vi "WireReadBlockDiagram.vi"(8 "error in":errorcluster, 10 "Terminal References":T3, 11 "State":T1={"paths"={"index cluster path"=path "C:/Users/bcelis.AMER/Documents/TBDCore/source/Utilities/Cluster to Tag Bus Scripts/Controls/IndexCluster.ctl", "cluster path"=path "C:/Users/bcelis.AMER/Documents/TBDCore/source/Utilities/Cluster to Tag Bus Scripts/Controls/SampleControl.ctl", "cluster to tag bus VI path"=path "C:/Users/bcelis.AMER/Documents/TBDCore/source/Utilities/Cluster to Tag Bus Scripts/ClustertoTagbus.vi", " tag bus to cluster VI path"=path ""}, "write VI ref"=refnum, "read VI ref"=refnum, "base cluster"=variant}) -> (0 "error out":errorcluster, 3 "State out":T1={"paths"={"index cluster path"=path "C:/Users/bcelis.AMER/Documents/TBDCore/source/Utilities/Cluster to Tag Bus Scripts/Controls/IndexCluster.ctl", "cluster path"=path "C:/Users/bcelis.AMER/Documents/TBDCore/source/Utilities/Cluster to Tag Bus Scripts/Controls/SampleControl.ctl", "cluster to tag bus VI path"=path "C:/Users/bcelis.AMER/Documents/TBDCore/source/Utilities/Cluster to Tag Bus Scripts/ClustertoTagbus.vi", " tag bus to cluster VI path"=path ""}, "write VI ref"=refnum, "read VI ref"=refnum, "base cluster"=variant})   [LabVIEW 2013]
uses:
  Controls/TerminalReferences.ctl
  Controls/StateCluster.ctl
  Controls/PathsCluster.ctl
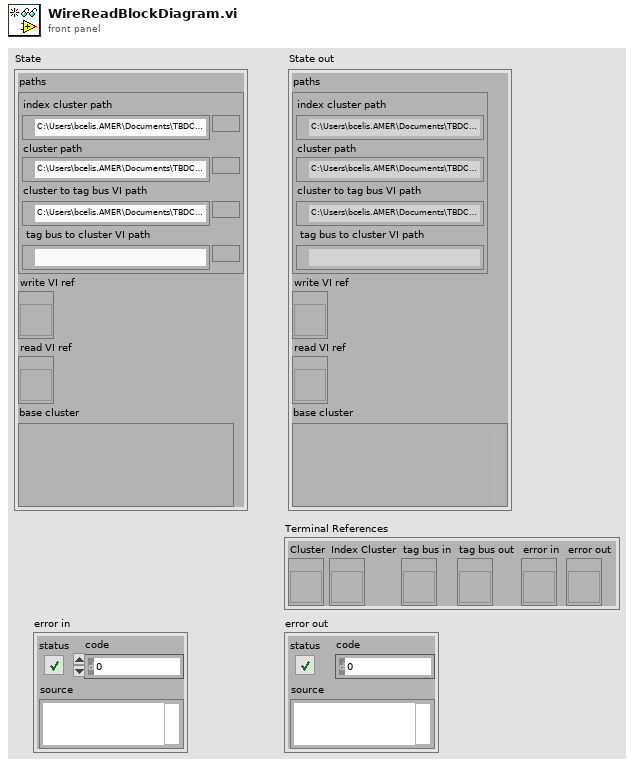
[diagram p1: front panel]
types:
  T1 = typedef "StateCluster.ctl" = cluster{"paths":T2, "write VI ref":refnum<vi>, "read VI ref":refnum<vi>, "base cluster":variant}
  T2 = typedef "PathsCluster.ctl" = cluster{"index cluster path":path, "cluster path":path, "cluster to tag bus VI path":path, " tag bus to cluster VI path":path}
  T3 = typedef "TerminalReferences.ctl" = cluster{"Cluster":refnum<vi>, "Index Cluster":refnum<vi>, "tag bus in":refnum<vi>, "tag bus out":refnum<vi>, "error in ":refnum<vi>, "error out":refnum<vi>}
  T4 = typedef "tag bus.lvlib/tag descriptor.lvclass/Data Type.ctl" = enum16{"Double", "Single", "I64", "I32", "I16", "I8", "U64", "U32", "U16", "U8", "Boolean", "String", "Array of Double", "Array of Single", "Array of I64", "Array of I32", "Array of I16", "Array of I8", "Array of U64", "Array of U32", "Array of U16", "Array of U8", "Array of Boolean", "Array of String"}
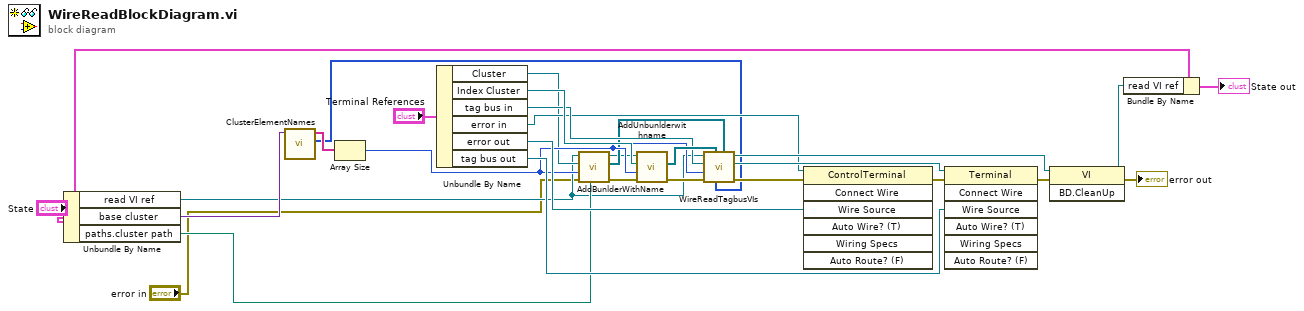
[diagram p0: block diagram]
diagram:
  n1 = Unbundle By Name("State") -> ("read VI ref"=w2:refnum<vi>, "base cluster"=w24:variant, "paths.cluster path"=w4:path)
  n2 = call "ClusterElementNames.vi"("input cluster"=w24) -> ("DataTypes"=w3:T4[], "Elements Names"=w23:string[])  [unwired: 8 in, 1 out]
  n3 = Array Size(array=w23) -> (size(s)=w9:i32)
  n4 = Unbundle By Name("Terminal References") -> ("Cluster"=w6:refnum<vi>, "Index Cluster"=w26:refnum<vi>, "tag bus in"=w19:refnum<vi>, "error in"=w12:refnum<vi>, "error out"=w14:refnum<vi>, "tag bus out"=w13:refnum<vi>)
  n5 = call "AddBunlderWithName.vi"("Cluster Path"=w4, "error in"="error in", "elements in cluster"=w9, "cluster terminal"=w6, "VI in"=w2) -> ("error out"=w5:errorcluster, "terminals"=w8:refnum<vi>[], "VI out"=w7:refnum<vi>)  [unwired: 4 in]
  n6 = call "AddUnbunlderwithname.vi"("error in"=w5, "elements in cluster"=w9, "cluster terminal"=w26, "VI in"=w7) -> ("error out"=w11:errorcluster, "terminals"=w25:refnum<vi>[])  [unwired: 5 in, 1 out]
  n7 = call "WireReadTagbusVIs.vi"("terminals data"=w8, "DataTypes"=w3, "terminals indexes"=w25, "error in"=w11, "elements in cluster"=w9, "tag bus in in"=w19, "VI in"=w2) -> ("error out"=w10:errorcluster, "tag bus out"=w15:refnum<vi>, "VI out"=w18:refnum<vi>)  [unwired: 2 in]
  n8 = invoke on="Invoke Node" class="ControlTerminal" method="Connect Wire"(reference=w12, error in=w10, "Wire Source"=w14) -> (error out=w17:errorcluster)  [unwired: 4 in, 6 out]
  n9 = invoke on="Invoke Node" class="Terminal" method="Connect Wire"(reference=w15, error in=w17, "Wire Source"=w13) -> (error out=w16:errorcluster)  [unwired: 4 in, 6 out]
  n10 = invoke class="VI" method="BD.CleanUp"(reference=w18, error in=w16) -> (reference out=w20:refnum<vi>, error out=→"error out":errorcluster)  [unwired: 1 in, 1 out]
  n11 = Bundle By Name(cluster="State", "read VI ref"=w20) -> (→"State out":T1)
